vi "Analyse Data.vi"(8 "error in":errorcluster, 11 "Data":dbl[][](array[numeric]) format="%0.2f") -> (0 "error out":errorcluster)   [LabVIEW 2021]
uses:
  <vilib>/Analysis/baseanly.llb/Mean (DBL).vi
  <vilib>/Analysis/NI_AALBase.lvlib
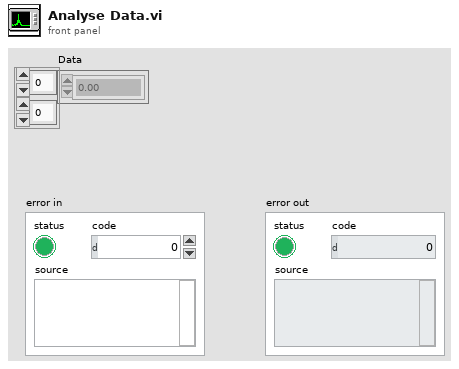
[diagram p1: front panel]
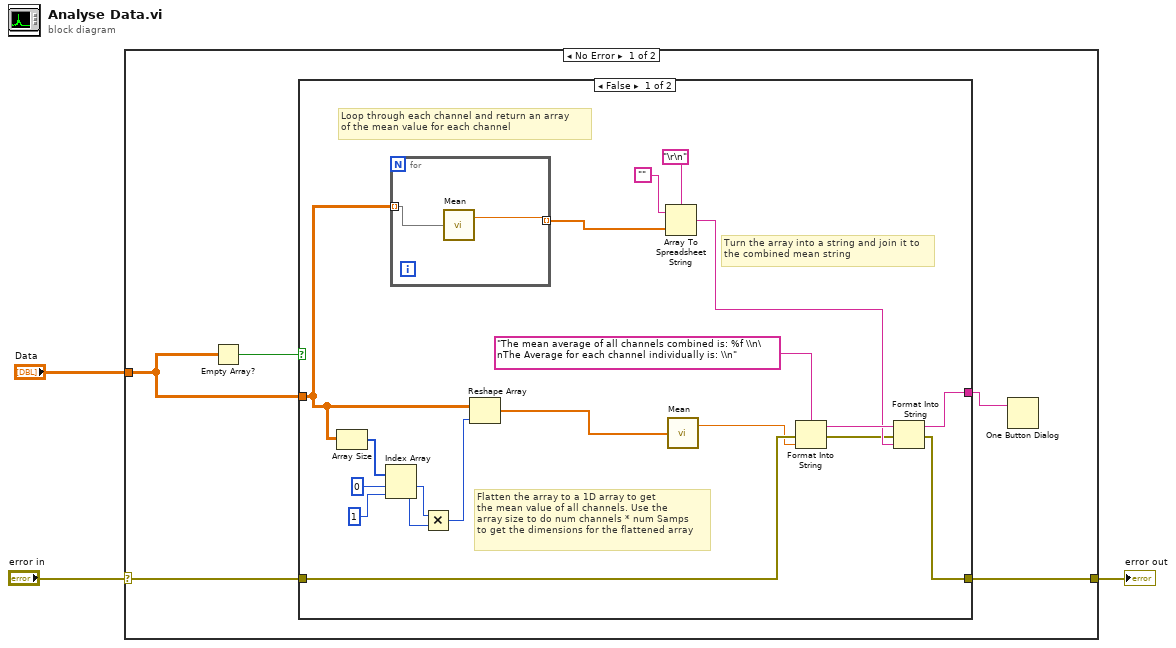
[diagram p0: block diagram]
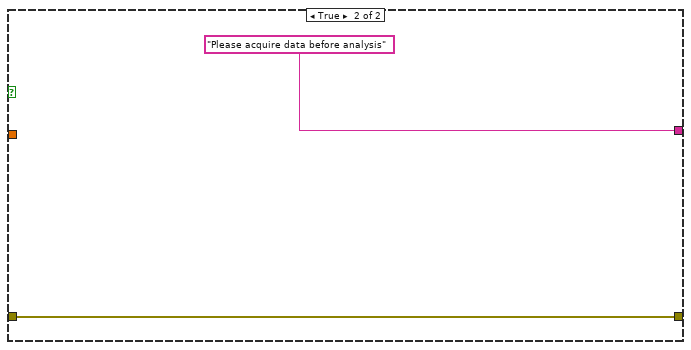
[diagram p2: hidden frame]
diagram:
  n1 = case shown="No Error" "error in" {
    selector: "error in" -> [w5 w32]
    tunnel: [w4 w32] -> w2
    tunnel: "Data" -> [w7 _]
    frame No Error {
      n2 = Empty Array?(array=w7) -> (empty?=w8:bool)
      n3 = case shown="False" w8 {
        tunnel: w7 -> [w17 _]
        tunnel: [w12 "Please acquire data before analysis"] -> w6
        tunnel: w5 -> [w27 w30]
        tunnel: [w9 w30] -> w4
        frame False {
          # "Turn the array into a string and join it to\nthe combined mean string"
          # "Loop through each channel and return an array\nof the mean value for each channel"
          # "Flatten the array to a 1D array to get\nthe mean value of all channels. Use the\narray size to do num channels * num Samps\nto get the dimensions for the flattened array"
          n4 = Array Size(array=w17) -> (size(s)=w23:i32[])
          n5 = Index Array "Index Array"(array=w23, index #1=0 ("index"), index #2=1 ("index")) -> (element #1=w20:i32, element #2=w19:i32)
          n6 = for {
            tunnel: w17 -> [w29] mode=indexing
            tunnel: [w28] -> w16 mode=indexing
            n7 = call-poly <vilib>:"Mean.vi"("X"=w29) -> ("mean"=w28:dbl)  [unwired: 1 out]
          }
          n8 = Multiply(x=w20, y=w19) -> (x*y=w18:i32)
          n9 = Reshape Array "Reshape Array"(w17, w18) -> (w24:dbl[])
          n10 = Array To Spreadsheet String(delimiter (Tab)="\r\n", array=w16, 3:"") -> (spreadsheet string=w13:string)
          n11 = call-poly <vilib>:"Mean.vi"("X"=w24) -> ("mean"=w25:dbl)  [unwired: 1 out]
          n12 = Format Into String(format string="The mean average of all channels combined is: %f \\n\nThe Average for each channel individually is: \\n", error in=w27, w25) -> (resulting string=w14:string, error out=w10:errorcluster)  [unwired: 1 in]
          n13 = Format Into String(initial string=w14, error in=w10, w13) -> (resulting string=w12:string, error out=w9:errorcluster)  [unwired: 1 in]
        }
        frame True {
        }
      }
      n14 = One Button Dialog(message=w6) -> ()  [unwired: 1 in, 1 out]
    }
    frame Error {
    }
  }
  "error out" <- w2
